vi "unit_read.vi"(4 "error in (no error)":errorcluster, 6 "Container State":T2, 7 "Display State In":T1={"calibration"=0.0, "unit"="m"}) -> (0 "error out":errorcluster, 2 "Value":string, 3 "Display State Out":T1={"calibration"=0.0, "unit"="m"})   [LabVIEW 2016, in "calibratedIOField.xctl"]
uses:
  calibratedIOField.xctl
  <vilib>/_xctls/Container State.ctl
  calibratedIOField_state.ctl
  <vilib>/_xctls/XControlSupport.lvlib
panel:
  # "Replace the Value Indicator below with an Indicator of desired type.\nDo not remove this Indicator or the others from the connector pane. \nDo not change the connector pane pattern.\nThe Value Indicator should always be the second terminal from top on the output side in the connector pane."
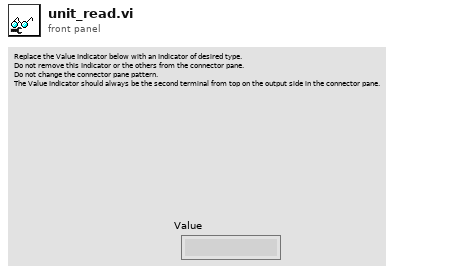
[diagram p1: front panel]
types:
  T1 = typedef "calibratedIOField.xctl/calibratedIOField_state.ctl" = cluster{"calibration":dbl, "unit":string}
  T2 = typedef "XControlSupport.lvlib/Container State.ctl" = cluster{"Indicator?":bool, "Run Mode?":bool, " Refnum":refnum<vi>}
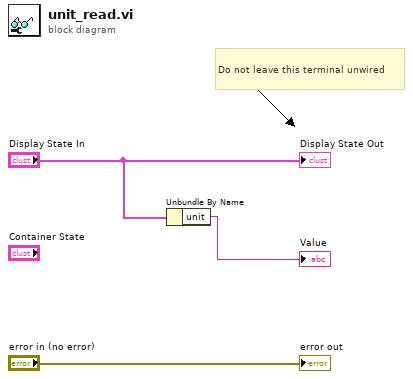
[diagram p0: block diagram]
diagram:
  # "Do not leave this terminal unwired"
  n1 = Unbundle By Name("Display State In") -> ("unit"=→"Value":string)
  "error out" <- "error in (no error)"
  "Display State Out" <- "Display State In"
